vi "printRC.vi"(10 "additional information":string, 11 "RC":i32) -> (0 "error out":T1)   [LabVIEW 2016]
doc: "Depending on the input \"RC\" (Return Code) this VI fills up the error out-Cluster with additional information about the emerged error. You can add additional information by typing it into the corresponding input (e.g. the function name where the error ocurred). The string will be added to the error description of the error-Cluster in brackets."
uses:
  Controls/Error_Out.ctl
  Files_ASC500/DLL/daisybase.dll
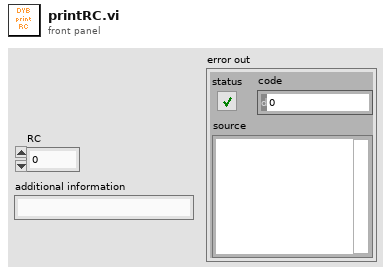
[diagram p1: front panel]
types:
  T1 = typedef "Error_Out.ctl" = errorcluster
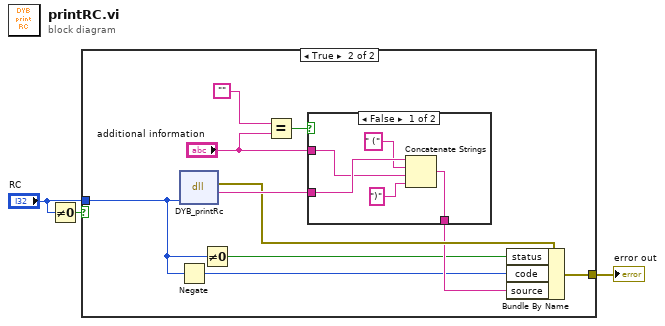
[diagram p0: block diagram]
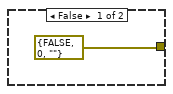
[diagram p2: hidden frame]
diagram:
  n1 = Not Equal To 0?(x="RC") -> (x != 0?=w3:bool)
  n2 = case shown="True" w3 {
    tunnel: "RC" -> [_ w10]
    tunnel: [errorcluster {FALSE, 0, ""} w5] -> w1
    frame False {
    }
    frame True {
      n3 = Negate(x=w10) -> (-x=w7:i32)
      n4 = dll-call lib="G:/SCMOperations/Share/ELE/Produkt Information/ASC500/04 Remote Control/02 development versions/2018Nov06/Files_ASC500/DLL/daisybase.dll" fn="DYB_printRc"("RC"=w10) -> (error out=w9:errorcluster, "return type"=w14:string)  [unwired: 4 in, 1 out]
      n5 = Not Equal To 0?(x=w10) -> (x != 0?=w6:bool)
      n6 = Equal?(x="", y="additional information") -> (x = y?=w12:bool)
      n7 = case shown="False" w12 {
        tunnel: w14 -> [w19 w20]
        tunnel: "additional information" -> [w16 _]
        tunnel: [w15 w20] -> w8
        frame False {
          n8 = Concatenate Strings(w19, " (" ("string"), w16, ")" ("string")) -> (w15:string)
        }
        frame True {
        }
      }
      n9 = Bundle By Name(cluster=w9, "status"=w6, "code"=w7, "source"=w8) -> (w5:errorcluster)
    }
  }
  "error out" <- w1
